vi "Initialize Uncompress FPGA (SubVI).vi"(11 "Data In":T1={"Image Height"=3072, "Image Width"=3072, "Frame Rate"=3072, "Movie File REF"=refnum, "Image REF"=refnum, "FPGA REF"=refnum}) -> (3 "Data Out":T1={"Image Height"=3072, "Image Width"=3072, "Frame Rate"=3072, "Movie File REF"=refnum, "Image REF"=refnum, "FPGA REF"=refnum})   [LabVIEW 2015]
uses:
  Common/Controls (HOST)/Replay Data Bundle.ctl
  <vilib>/vision/Image Controls.llb/IMAQ Image.ctl
  <vilib>/FPGAPlugInAG/Dynamic/niLvFpga_Reset_Dynamic.vi
  <vilib>/rvi/interface/common/niFpgaWaitOnOcc.vi
  <vilib>/Utility/error.llb/Error Cluster From Error Code.vi
  <vilib>/rvi/errors/niLvFpgaAdjustHostInterfaceError.vi
  <vilib>/FPGAPlugInAG/Dynamic/niLvFpga_Run_Dynamic.vi
  <vilib>/rvi/interface/nirviMethod/nirviMethod.xnode
  <vilib>/rvi/interface/nirviReadWriteControl/nirviReadWriteControl.xnode
  <vilib>/FPGAPlugInAG/Dynamic/niLvFpga_ConfigureFifo_Dynamic.vi
  <vilib>/rvi/errors/niLvFpgaMergeErrorWithErrorCode.vi
  <vilib>/FPGAPlugInAG/Dynamic/niLvFpga_StartFifo_Dynamic.vi
  NiFpgaLv.dll
  <vilib>/rvi/interface/Simulation/niFpgaSimulationCallBeginRW.vi
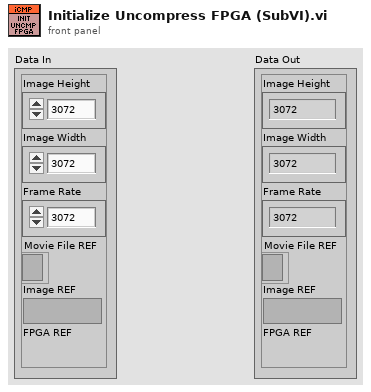
[diagram p1: front panel]
types:
  T1 = typedef "Replay Data Bundle.ctl" = cluster{"Image Height":i32, "Image Width":i32, "Frame Rate":i32, "Movie File REF":refnum<file>, "Image REF":T2, "FPGA REF":refnum<k20>}
  T2 = typedef "IMAQ Image.ctl" = refnum<image>
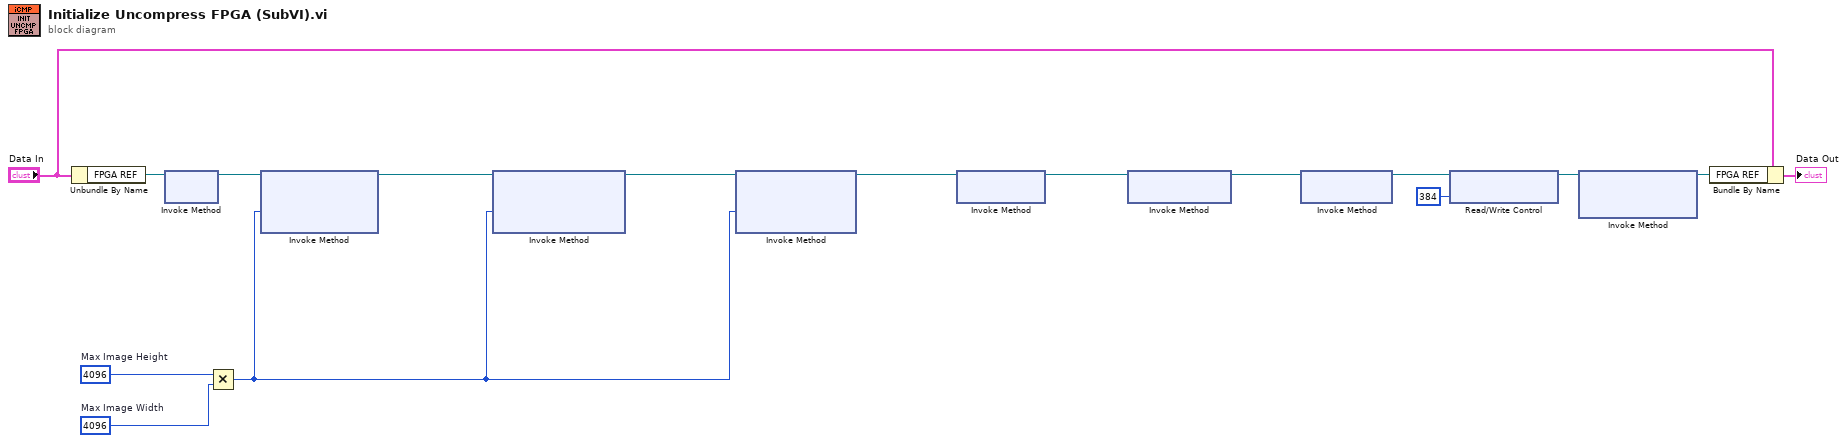
[diagram p0: block diagram]
diagram:
  w12 = u32 4096  # Max Image Width
  w13 = u32 4096  # Max Image Height
  n1 = Unbundle By Name("Data In") -> ("FPGA REF"=w4:refnum<k20>)
  n2 = xnode "Invoke Method"("FPGA VI Reference In"=w4) -> ("FPGA VI Reference Out"=w7:refnum<k20>)  [unwired: 1 in, 1 out]
  n3 = Multiply(x=w13, y=w12) -> (x*y=w11:u32)
  n4 = xnode "Invoke Method"("FPGA VI Reference In"=w7, "Requested Depth"=w11) -> ("FPGA VI Reference Out"=w16:refnum<k20>)  [unwired: 1 in, 2 out]
  n5 = xnode "Invoke Method"("FPGA VI Reference In"=w16, "Requested Depth"=w11) -> ("FPGA VI Reference Out"=w15:refnum<k20>)  [unwired: 1 in, 2 out]
  n6 = xnode "Invoke Method"("FPGA VI Reference In"=w15, "Requested Depth"=w11) -> ("FPGA VI Reference Out"=w14:refnum<k20>)  [unwired: 1 in, 2 out]
  n7 = xnode "Invoke Method"("FPGA VI Reference In"=w14) -> ("FPGA VI Reference Out"=w9:refnum<k20>)  [unwired: 1 in, 1 out]
  n8 = xnode "Invoke Method"("FPGA VI Reference In"=w9) -> ("FPGA VI Reference Out"=w10:refnum<k20>)  [unwired: 1 in, 1 out]
  n9 = xnode "Invoke Method"("FPGA VI Reference In"=w10) -> ("FPGA VI Reference Out"=w8:refnum<k20>)  [unwired: 1 in, 1 out]
  n10 = xnode "Read/Write Control"("FPGA VI Reference In"=w8, "Image Width (/8)"=u16 384 ("Image Width")) -> ("FPGA VI Reference Out"=w6:refnum<k20>)  [unwired: 1 in, 1 out]
  n11 = xnode "Invoke Method"("FPGA VI Reference In"=w6) -> ("FPGA VI Reference Out"=w2:refnum<k20>)  [unwired: 2 in, 1 out]
  n12 = Bundle By Name(cluster="Data In", "FPGA REF"=w2) -> (→"Data Out":T1)
